vi "Get Status.vi"(8 "error in (no error)":errorcluster, 11 "PicoScope 3000a in":refnum<class "PicoScope 3000a.lvclass">) -> (0 "error out":errorcluster, 2 "Status Array":bool[](array[boolean]), 3 "PicoScope 3000a out":refnum<class "PicoScope 3000a.lvclass">)   [LabVIEW 2018, in "PicoScope 3000a.lvlib" / "PicoScope 3000a.lvclass"]
doc: "This Override method is used to get the Oscope instrument status. The status data MUST be formatted into the 'Status Array' indicator as 1D array of boolean data ."
uses:
  PicoScope 3000a.lvclass
  PicoScope 3000a.lvclass/PicoScope 3000a.ctl
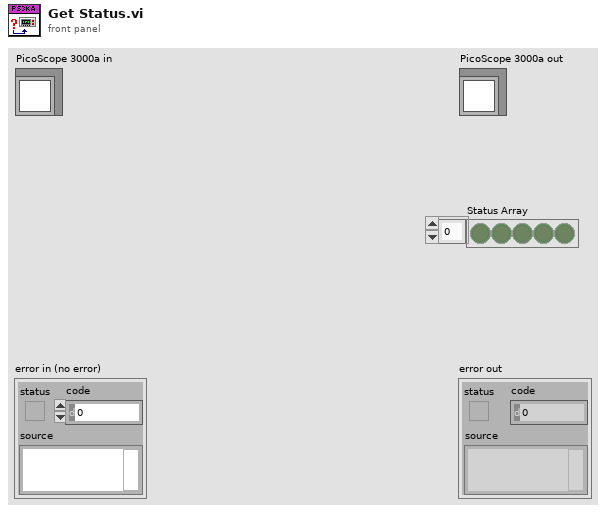
[diagram p1: front panel]
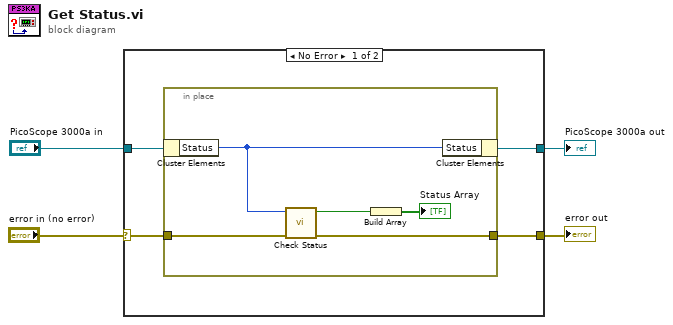
[diagram p0: block diagram]
diagram:
  n1 = case shown="No Error" "error in (no error)" {
    selector: "error in (no error)" -> [w7 w14]
    tunnel: "PicoScope 3000a in" -> [w8 w15]
    tunnel: [w6 w14] -> w2
    tunnel: [w5 w15] -> w1
    frame No Error {
      n2 = in-place {
        in-place-border: w7 -> [w12]
        in-place-border: [w9] -> w6
        n3 = in-place-cluster #1(w8) -> ("Status"=w13:i32)
        n4 = call "Check Status.vi"("error in (no error)"=w12, "Status Code"=w13) -> ("error out"=w9:errorcluster, "Error?"=w11:bool)  [unwired: 8 in]
        n5 = Build Array(w11) -> (→"Status Array":bool[])
        n6 = in-place-cluster #1("Status"=w13) -> (w5:refnum<class "PicoScope 3000a.lvclass">)
      }
    }
    frame Error {
    }
  }
  "error out" <- w2
  "PicoScope 3000a out" <- w1
